vi "Open.vi"   [LabVIEW 2014, in "LMH-LINX.lvlib"]
doc: "Open a connection to a remote LINX device or the local I/O of a LINX device."
uses:
  <vilib>/MakerHub/LINX/LMH-LINX.lvlib
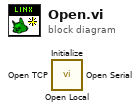
[diagram p0: block diagram]
diagram:
  n1 = call <vilib>:"Open Local.vi"() -> ()  [unwired: 9 in, 3 out]
  n2 = call <vilib>:"Initialize.vi"() -> ()  [unwired: 9 in, 3 out]
  n3 = call <vilib>:"Open TCP.vi"() -> ()  [unwired: 9 in, 3 out]
  n4 = call <vilib>:"Open Serial.vi"() -> ()  [unwired: 9 in, 3 out]
